vi "GFITS_toImstats.vi"(6 "wait":i32, 7 "nelems":u32, 8 "error in (no error)":errorcluster, 9 "ptr":u64, 10 "cmd":string) -> (0 "error out":errorcluster, 2 "resp":string)   [LabVIEW 2016]
uses:
  DBSHAND/private/vis/DatabaseHand_Element_Get(bool).vi
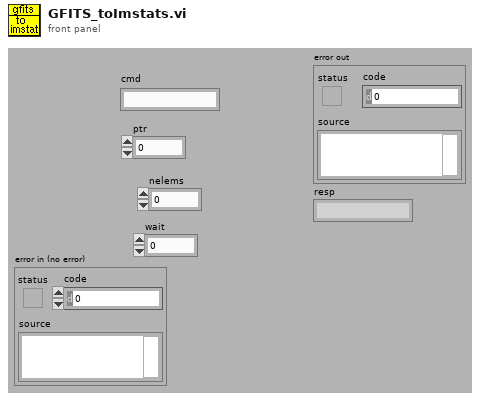
[diagram p1: front panel]
types:
  T1 = typedef "DatabaseHand_RefNum.ctl" = refnum<vi>
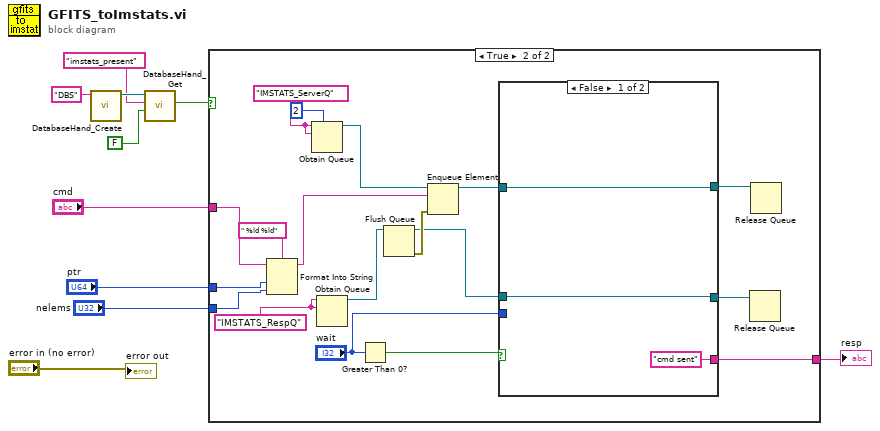
[diagram p0: block diagram]
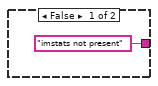
[diagram p2: hidden frame]
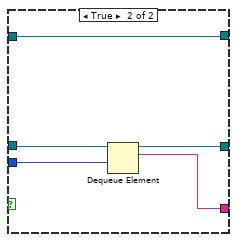
[diagram p3: hidden frame]
diagram:
  n1 = call "DatabaseHand_Create.vi"("Name"="DBS") -> ("Database RefNum out"=w9:T1)  [unwired: 1 in, 9 out]
  n2 = call-poly "DatabaseHand_Get.vi"("default value"=FALSE, "name"="imstats_present" ("default value"), "Database RefNum in"=w9) -> ("value"=w6:bool)  [unwired: 2 in, 6 out]
  n3 = case shown="True" w6 {
    tunnel: "cmd" -> [_ w25]
    tunnel: "ptr" -> [_ w26]
    tunnel: ["imstats not present" ("name (unnamed)") w13] -> w2
    tunnel: "nelems" -> [_ w12]
    frame False {
    }
    frame True {
      w19 = "IMSTATS_RespQ" ("name (unnamed)")
      w29 = "IMSTATS_ServerQ" ("name (unnamed)")
      n4 = Format Into String(format string=" %ld %ld", initial string=w25, w26, w12) -> (resulting string=w23:string)  [unwired: 1 in, 1 out]
      n5 = Obtain Queue(max queue size (-1, unlimited)=2, name (unnamed)=w29, element data type=w29) -> (queue out=w28:refnum<queue>)  [unwired: 2 in, 2 out]
      n6 = Obtain Queue(name (unnamed)=w19, element data type=w19) -> (queue out=w18:refnum<queue>)  [unwired: 3 in, 2 out]
      n7 = Greater Than 0?(x="wait") -> (x > 0?=w22:bool)
      n8 = Flush Queue(queue=w18) -> (queue out=w16:refnum<queue>, error out=w17:errorcluster)  [unwired: 1 in, 1 out]
      n9 = Enqueue Element(queue=w28, element=w23, error in (no error)=w17) -> (queue out=w21:refnum<queue>)  [unwired: 3 out]
      n10 = case shown="False" w22 {
        tunnel: w21 -> [w32 w37]
        tunnel: [w32 w37] -> w20
        tunnel: w16 -> [w31 w36]
        tunnel: "wait" -> [_ w35]
        tunnel: [w31 w34] -> w14
        tunnel: ["cmd sent" ("name (unnamed)") w33] -> w13
        frame False {
        }
        frame True {
          n11 = Dequeue Element(queue=w36, timeout in ms (-1)=w35) -> (queue out=w34:refnum<queue>, element=w33:string)  [unwired: 1 in, 2 out]
        }
      }
      n12 = Release Queue(queue=w14) -> ()  [unwired: 1 in, 4 out]
      n13 = Release Queue(queue=w20) -> ()  [unwired: 1 in, 4 out]
    }
  }
  "resp" <- w2
  "error out" <- "error in (no error)"
